vi "Main.vi"() -> ()   [LabVIEW 2026]
doc: "This Continuous Measurement sample project is based on the Queued Message Handler template.\n\nThe Event Handling Loop generates messages based on user interface actions.\n\nThe Message Handling Loop processes messages generated by the Event Handling Loop, or by other messages. There are also Acquisition and Logging message handling loop subVIs, and a chart updating loop."
uses:
  controls/Messaging Payloads/Sensor CoreData.ctl
  controls/Messaging Payloads/Sensor CoreData Cluster.ctl
  controls/UI/Units Enum.ctl
  controls/UI/Signal Enum.ctl
  controls/UI/Settings Cluster.ctl
  controls/UI/Acq Settings.ctl
  Acquisition/Instrument Specifications Configuration.ctl
  Acquisition/Instrument Specifications Cluster Configuration.ctl
  controls/UI/Measurement Role.ctl
  controls/UI/Config Settings.ctl
  Processing/Processing Settings.ctl
  Processing/Test Parameters.ctl
  Processing/Test Parameters Cluster.ctl
  controls/UI/Test Sequence Context.ctl
  controls/UI/Direction.ctl
  controls/UI/Session Identfiers.ctl
  controls/UI/Test Sequence Settings.ctl
  controls/UI/Test Sequence State.ctl
  controls/UI/Test Sequence Enum.ctl
  controls/Controller/Stimulus Settings.ctl
  controls/Controller/Stimulus Outputs.ctl
  controls/Controller/Stimulus Output.ctl
  controls/Controller/Controller Core Data.ctl
  controls/Controller/Stimulus Output Configuration.ctl
  controls/Controller/Stimulus Role.ctl
  controls/UI/UI Data.ctl
  controls/UI/UI State.ctl
  controls/UI/System Config.ctl
  controls/UI/Analog Output.ctl
  controls/UI/UUT Display Data.ctl
  Acquisition/Acquisition Payload.ctl
  Acquisition/Acquisition Context.ctl
  support/Architecture/Message Queue/Enqueue Message (Single).vi
  support/Architecture/Message Queue/Enqueue Message (Array).vi
  <vilib>/Utility/error.llb/Error Cluster From Error Code.vi
  <vilib>/ErrorRing/Error Ring.xnode
  support/Architecture/User Event - Stop/User Event - Stop.lvlib
  support/Architecture/Message Queue/Message Queue.lvlib
  Settings/Settings Dialog.vi
  Settings/Settings.lvlib
  Database/Database.lvlib
  Logging/Logging.lvlib
  Processing/Processing_Engine.lvlib
  Acquisition/Acquisition.lvlib
  support/UI Utilities/Login.vi
  Admin/Admin.lvlib
  Analysis/Analysis Dialog.vi
  Analysis/Analysis.lvlib
panel:
  in  "Manage Serial Numbers":bool
  in  "Simulation Mode":bool
  in  "Stop":bool
  in  "Start":bool
  out "Sensor Information":T1
  in  "Generate Analytics":bool
  out "Data":waveform(dbl)[](graph)
  in  "Settings":bool
  out "Status":string
  in  "Exit":bool
  # "Live Data"
  # "Test Control"
  # "ON"
  # "Automated Calibration & Test System\nMulti-Sensor Instrument Calibration Platform"
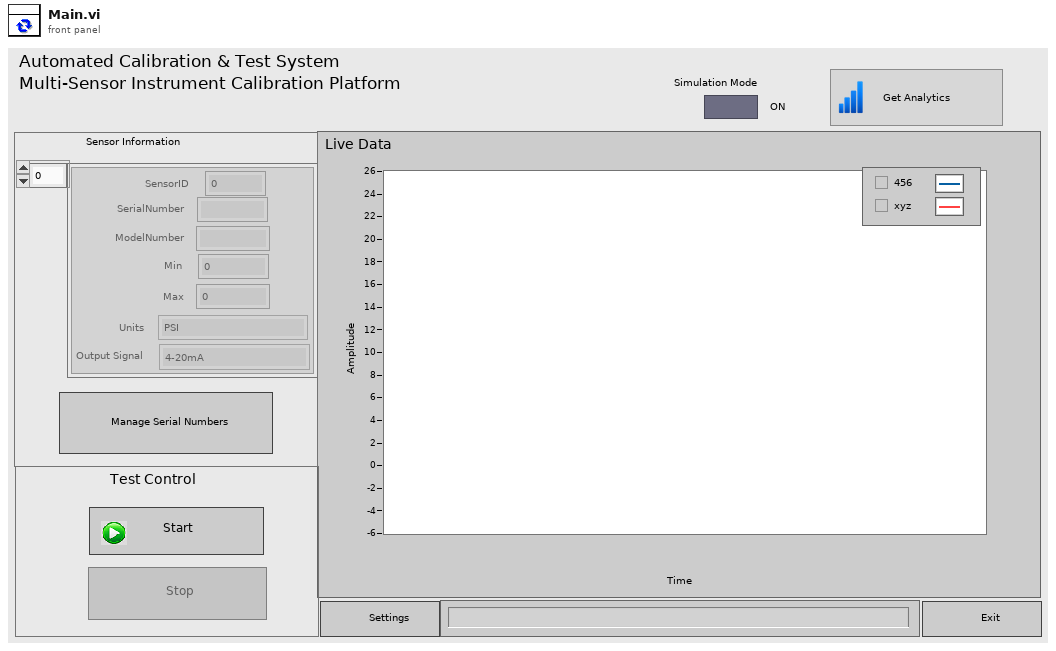
[diagram p1: front panel]
types:
  T1 = typedef "Sensor CoreData.ctl" = T2[]
  T2 = typedef "Settings.lvlib/Sensor CoreData Cluster.ctl" = cluster{"SerialNumber":string, "ModelNumber":string, "Min":dbl, "Max":dbl, "Units":T3, "Output Signal":T4, "SensorID":i32}
  T3 = typedef "Units Enum.ctl" = enum16{"PSI", "Deg C", "kPa", "GPM"}
  T4 = typedef "Signal Enum.ctl" = enum16{"4-20mA", "0-10V", "Thermocouple Type K"}
  T5 = typedef "UUT Display Data.ctl" = cluster{"Waveforms":waveform(dbl)[], "SensorIDs":i32[]}
  T6 = typedef "System Config.ctl" = cluster{"AdminHash":string, "LogFileBasePath ":path, "Config Settings":T7, "AnalogOutput":T8}
  T7 = typedef "Config Settings.ctl" = cluster{"Simulated Sensor Injection":dbl, "Base Device Name":string, "Simulation Mode":string}
  T8 = typedef "Settings.lvlib/Analog Output.ctl" = cluster{"Pressure Controller":string, "Temperature Controller":string}
  T9 = typedef "UI State.ctl" = enum16{"Idle", "Acquiring and Logging", "Waiting for Exit", "Waiting for Exit (Acq Stopped)", "Waiting for Exit (Log Stopped)", "Waiting for Stop", "Waiting for Stop (Acq Stopped)", "Waiting for Stop (Log Stopped)"}
  T10 = typedef "UI Data.ctl" = cluster{"Start Ref":refnum<vi>, "Stop Ref":refnum<vi>, "Settings Ref":refnum<vi>, "Exit Ref":refnum<vi>, "Status Ref":refnum<vi>, "Data Ref":refnum<vi>, "Sim  Refnum":refnum<vi>}
  T11 = typedef "Settings Cluster.ctl" = cluster{"Acq Settings":T12, "Processing Settings":T16, "Session Identifiers":T21, "Test Sequence Settings":T22, "Stimulus Settings":T25}
  T12 = typedef "Acq Settings.ctl" = cluster{"Instrument Specifications":T13, "Config Settings":T7}
  T13 = typedef "Acquisition.lvlib/Instrument Specifications Configuration.ctl" = T14[]
  T14 = typedef "Acquisition.lvlib/Instrument Specifications Cluster Configuration.ctl" = cluster{"Sensor ID *":i32, "Target Sample Rate (Hz) *":dbl, "Steady-State Duration (s) *":i32, "Allowed Tolerance (%) FS *":dbl, "Max Settling Timeout (s) *":i32, "Physical Channel":string, "Measurement Role":T15}
  T15 = typedef "Settings.lvlib/Measurement Role.ctl" = enum16{"Reference", "UUT"}
  T16 = typedef "Processing_Engine.lvlib/Processing Settings.ctl" = cluster{"Sensor CoreData":T1, "Test Parameters":T17, "Measurement Roles":T15[], "Test Sequence Context":T19}
  T17 = typedef "Processing_Engine.lvlib/Test Parameters.ctl" = T18[]
  T18 = typedef "Settings.lvlib/Test Parameters Cluster.ctl" = cluster{"Steady-State Duration (s)":i32, "Allowed Tolerance (%) FS":dbl, "Max Settling Timeout (s)":i32}
  T19 = typedef "Settings.lvlib/Test Sequence Context.ctl" = cluster{"Direction":T20, "Cycle Number":i32, "Setpoint":dbl}
  T20 = typedef "Settings.lvlib/Direction.ctl" = enum16{"Acsending", "Descending"}
  T21 = typedef "Session Identfiers.ctl" = cluster{"SerialNumber":string[], "OperatorName":string}
  T22 = typedef "Test Sequence Settings.ctl" = cluster{"Test Sequence State":T23}
  T23 = typedef "Settings.lvlib/Test Sequence State.ctl" = cluster{"Test Sequence Enum":T24, "Point Index":i32, "Current Target":dbl, "Previous Target":dbl, "Simulation?":bool, "Direction":T20, "Transition Active?":bool, "Cycle Number":i32}
  T24 = typedef "Test Sequence Enum.ctl" = enum16{"Idle", "Start Point", "Point Complete", "Test Complete", "Abort Test", "Reset"}
  T25 = typedef "Settings.lvlib/Stimulus Settings.ctl" = cluster{"Stimulus Outputs":T26}
  T26 = typedef "Settings.lvlib/Stimulus Outputs.ctl" = T27[]
  T27 = typedef "Settings.lvlib/Stimulus Output.ctl" = cluster{"Controller Core Data":T28, "Stimulus Output Configuration":T29}
  T28 = typedef "Settings.lvlib/Controller Core Data.ctl" = cluster{"Min":dbl, "Max":dbl, "Units":T3, "Input Signal Type":T4, "Input Signal Min":dbl, "Input Signal Max":dbl}
  T29 = typedef "Settings.lvlib/Stimulus Output Configuration.ctl" = cluster{"DAQmx AO Physical Channel":tag, "Role":T30, "Model Numbers":string, "Serial Numbers":string, "Row":i32}
  T30 = typedef "Stimulus Role.ctl" = enum16{"Pressure Controller", "Temperature Controller"}
  T31 = typedef "Message Queue.lvlib/All Message Queues.ctl" = cluster{"UI":refnum<queue>, "Database":refnum<queue>, "Processing":refnum<queue>, "Acquisition":refnum<queue>, "Logging":refnum<queue>, "Analysis":refnum<queue>}
  T32 = enum8{"Enabled", "Disabled", "Disabled and Grayed Out"}
  T33 = typedef "Acquisition.lvlib/Acquisition Payload.ctl" = cluster{"Acq Settings":T12, "Acquisition Context":T34, "Stimulus Settings":T25}
  T34 = typedef "Acquisition.lvlib/Acquisition Context.ctl" = cluster{"Setpoint":dbl, "Previous Setpoint":dbl, "Transition Start Time":dbl, "Transition Active?":bool, "Acknowledgement Pending?":bool}
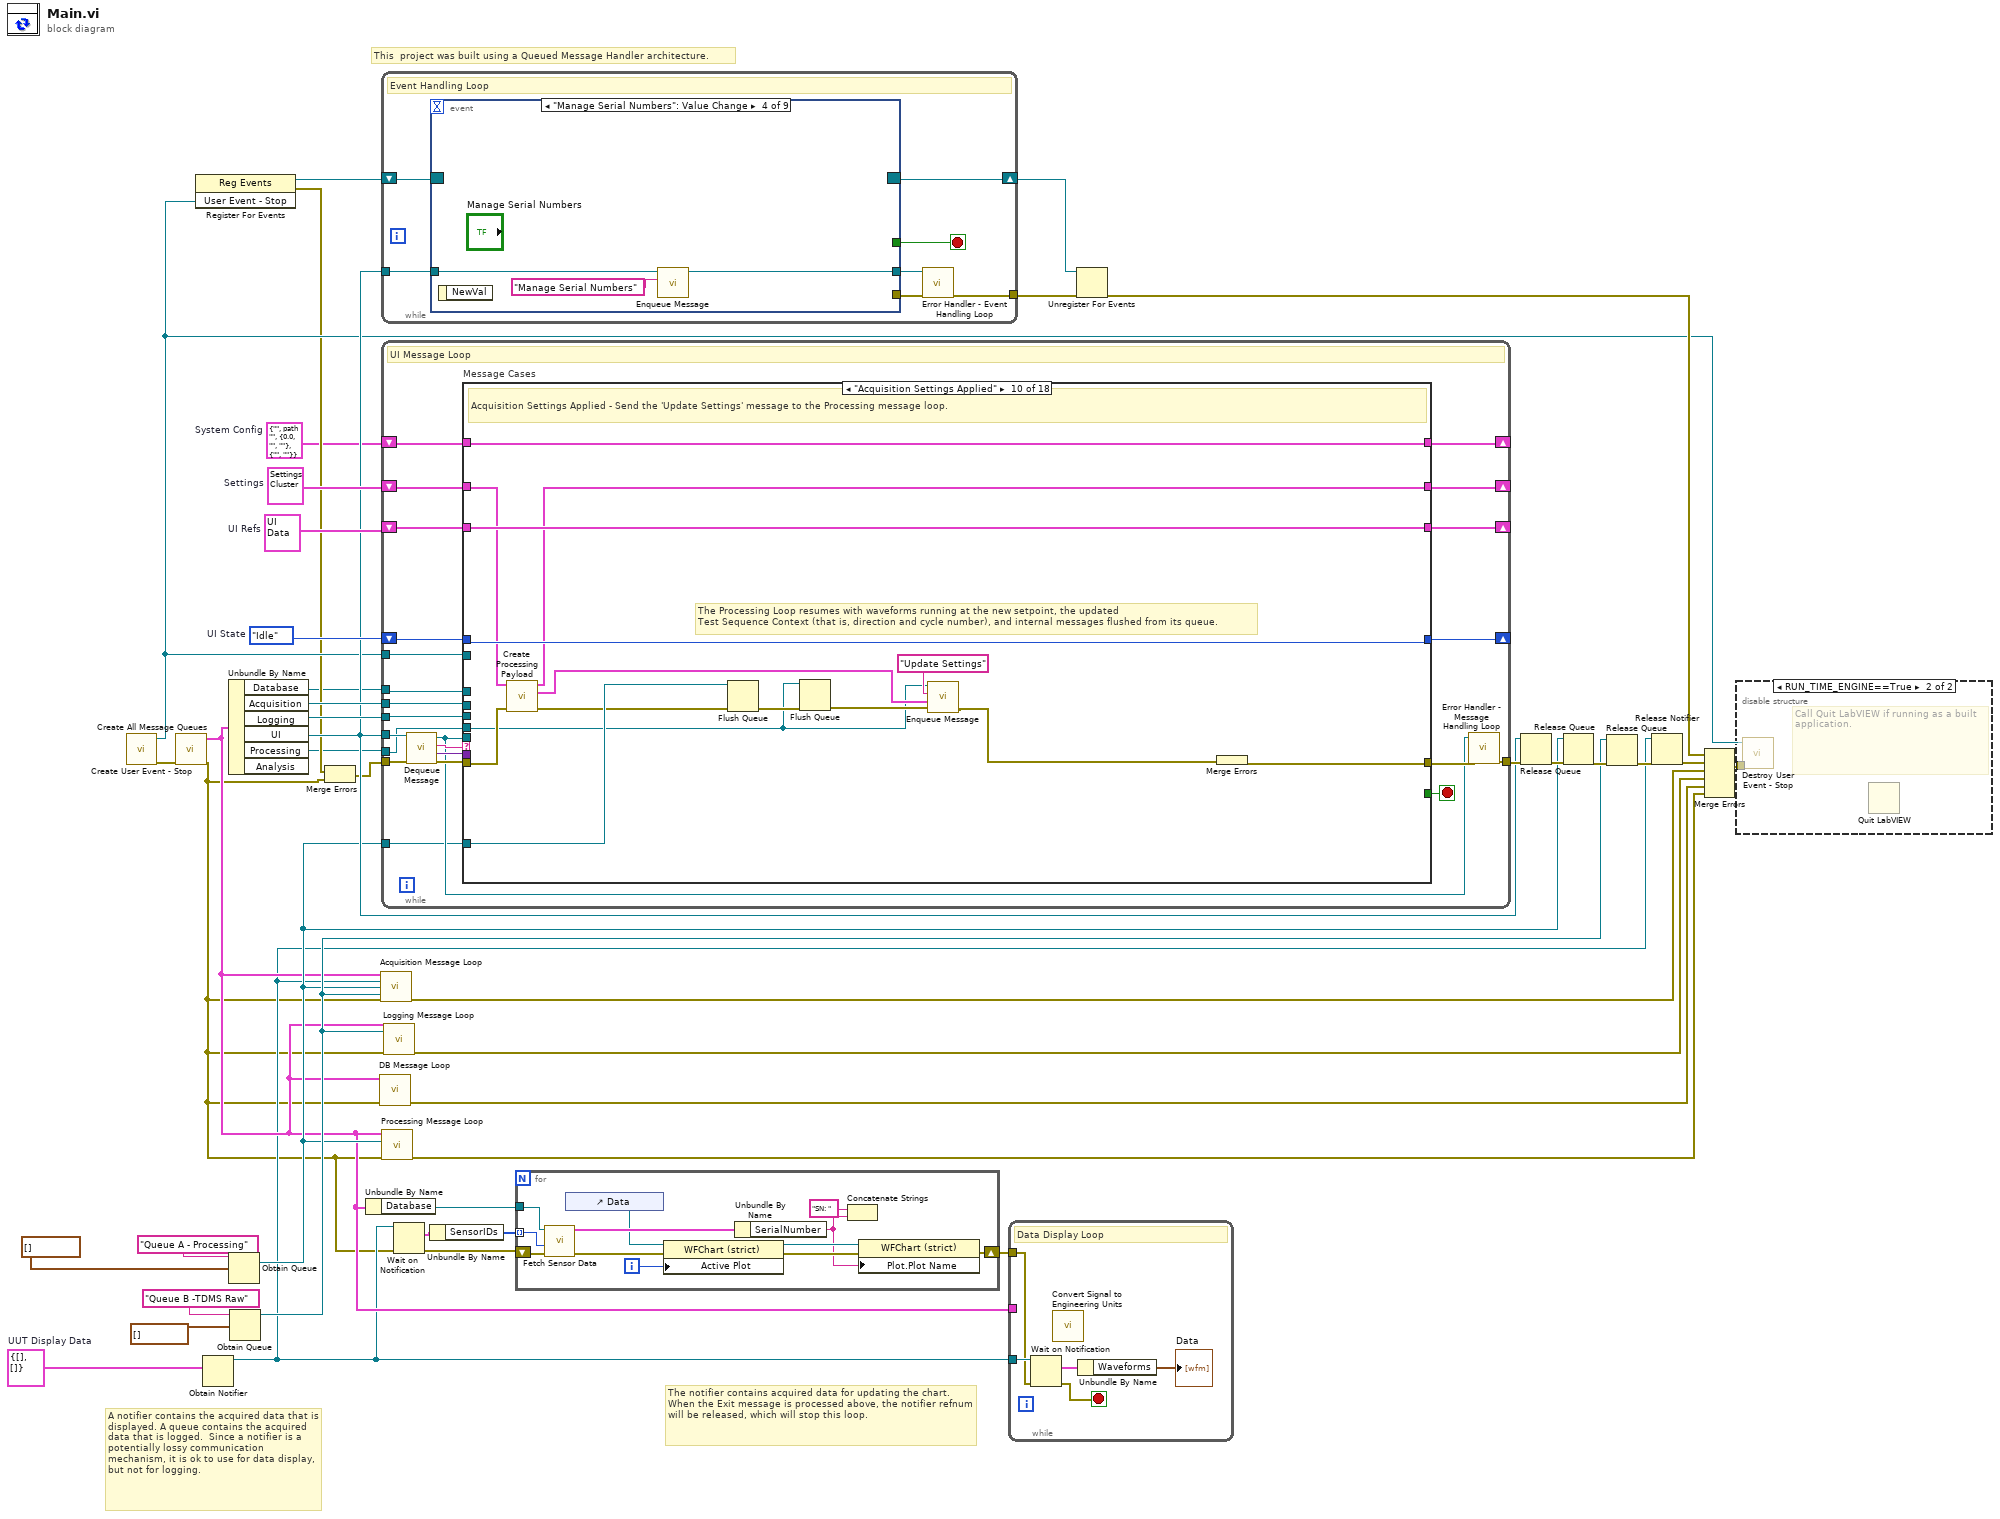
[diagram p0: block diagram]
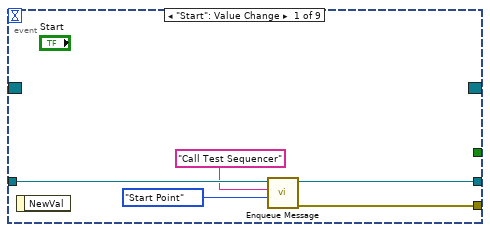
[diagram p3: hidden frame]
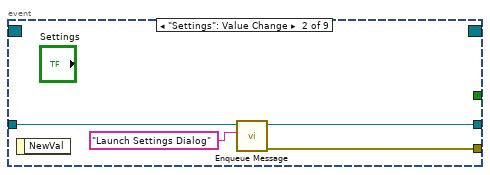
[diagram p4: hidden frame]
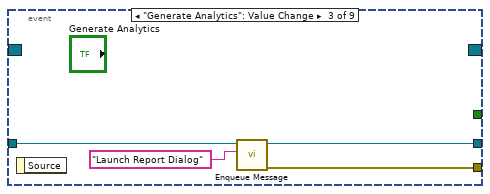
[diagram p5: hidden frame]
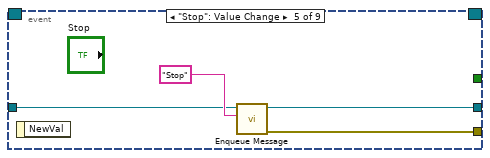
[diagram p6: hidden frame]
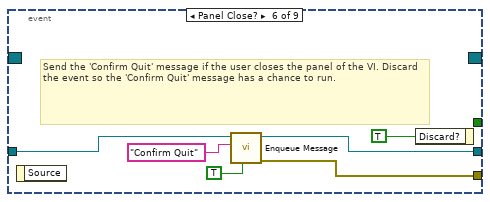
[diagram p7: hidden frame]
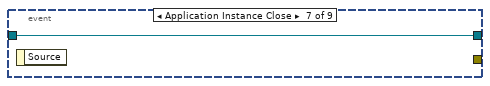
[diagram p8: hidden frame]
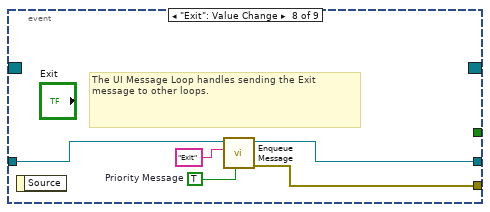
[diagram p9: hidden frame]
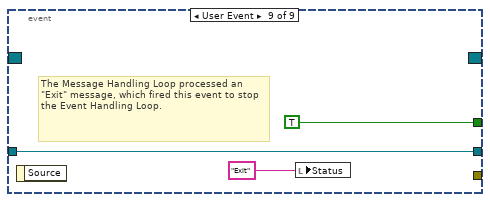
[diagram p10: hidden frame]
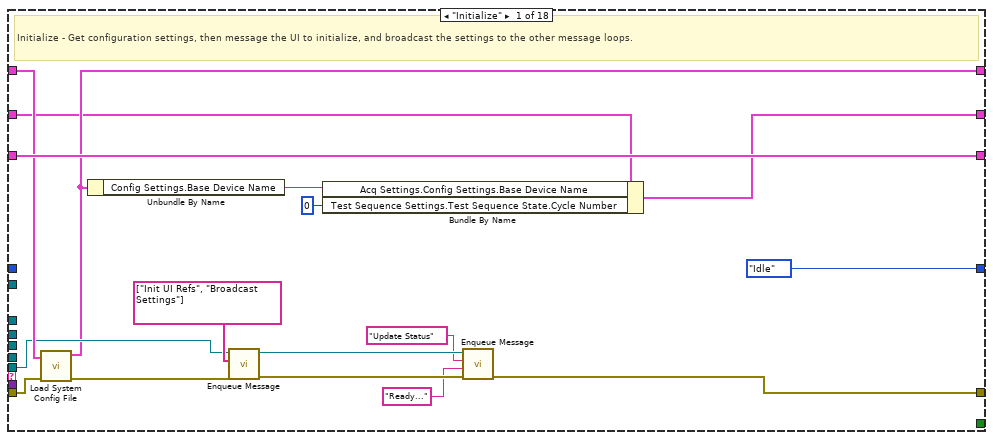
[diagram p11: hidden frame]
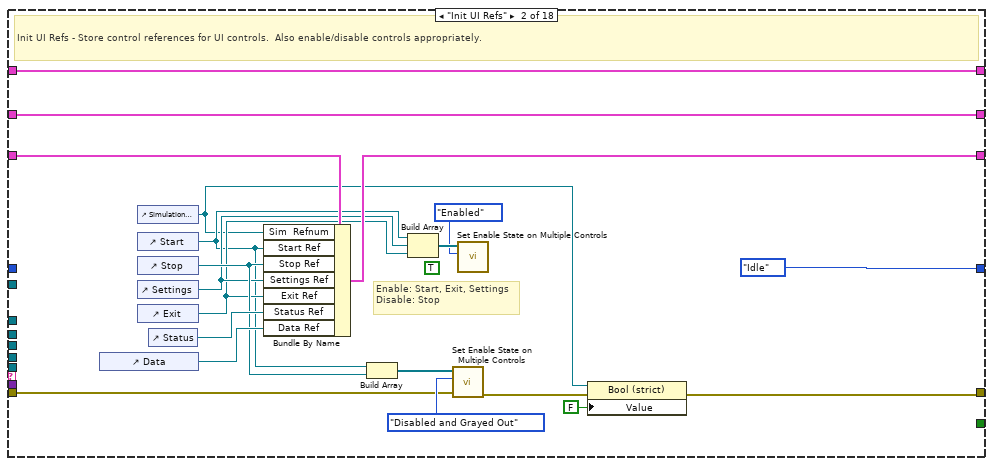
[diagram p12: hidden frame]
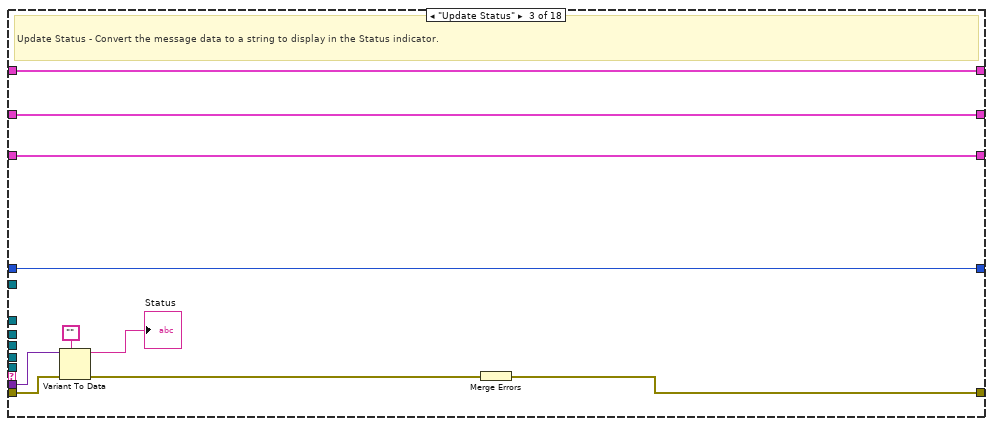
[diagram p13: hidden frame]
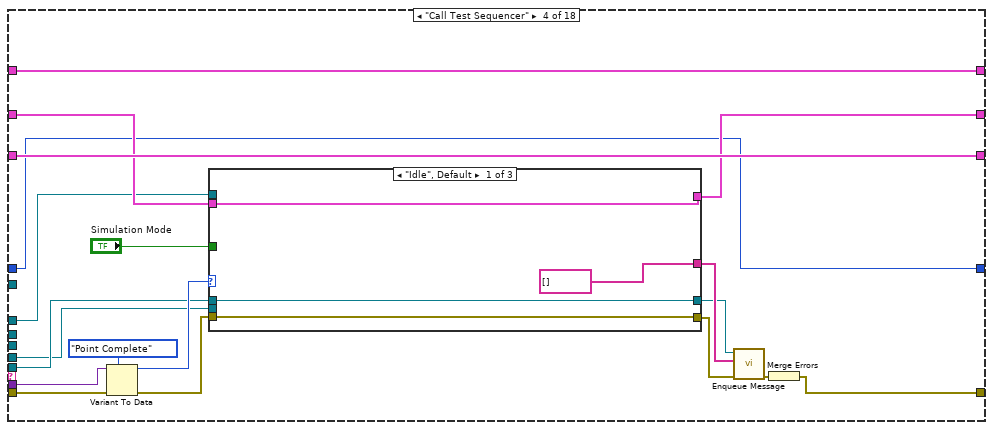
[diagram p14: hidden frame]
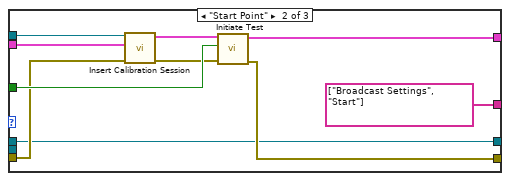
[diagram p15: hidden frame]
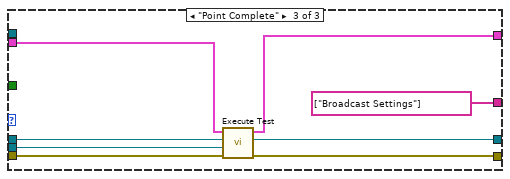
[diagram p16: hidden frame]
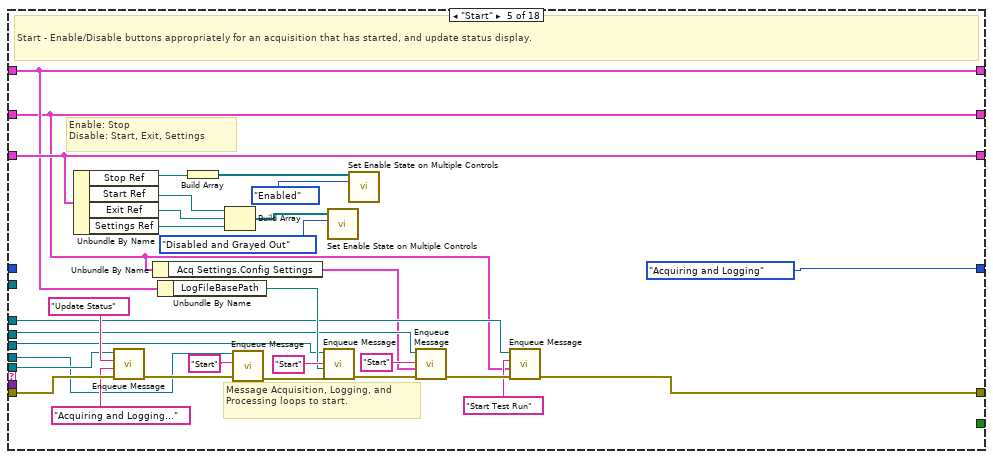
[diagram p17: hidden frame]
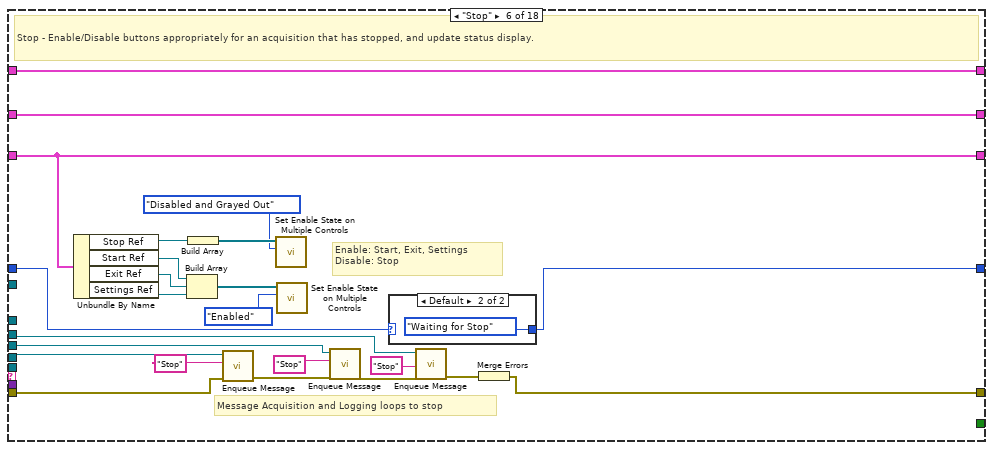
[diagram p18: hidden frame]
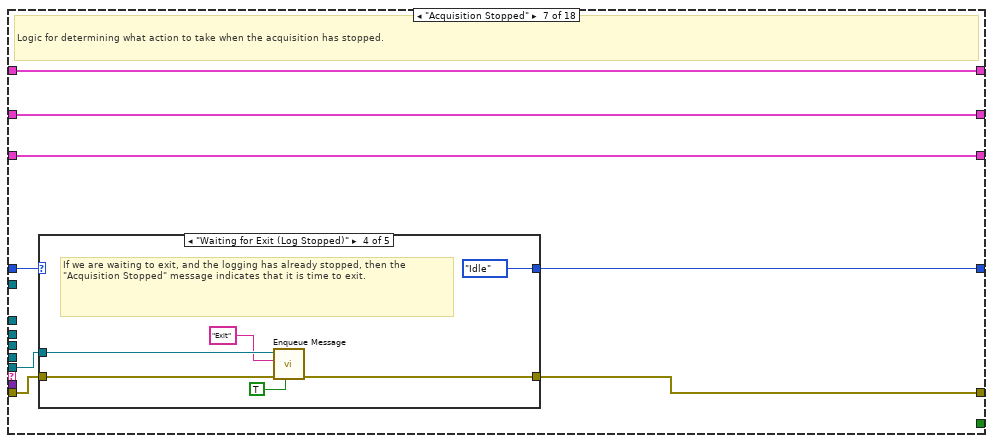
[diagram p20: hidden frame]
diagram:
  w9 = T5 {"Waveforms"=[], "SensorIDs"=[]}  # UUT Display Data
  w20 = T6 {"AdminHash"="", "LogFileBasePath "=path "", "Config Settings"={"Simulated Sensor Injection"=0.0, "Base Device Name"="", "Simulation Mode"=""}, "AnalogOutput"={"Pressure Controller"="", "Temperature Controller"=""}}  # System Config
  w32 = UI_State."Idle"  # UI State
  w35 = T10 {"Start Ref"=refnum, "Stop Ref"=refnum, "Settings Ref"=refnum, "Exit Ref"=refnum, "Status Ref"=refnum, "Data Ref"=refnum, "Sim  Refnum"=refnum}  # UI Refs
  w38 = T11 {"Acq Settings"={"Instrument Specifications"=[], "Config Settings"={"Simulated Sensor Injection"=0.0, "Base Device Name"="", "Simulation Mode"=""}}, "Processing Settings"={"Sensor CoreData"=[], "Test Parameters"=[], "Measurement Roles"=[], "Test Sequence Context"={"Direction"=enum."Acsending", "Cycle Number"=0, "Setpoint"=0.0}}, "Session Identifiers"={"SerialNumber"=[], "OperatorName"=""}, "Test Sequence Settings"={"Test Sequence State"={"Test Sequence Enum"=enum."Idle", "Point Index"=0, "Current Target"=0.0, "Previous Target"=0.0, "Simulation?"=FALSE, "Direction"=enum."Acsending", "Transition Active?"=FALSE, "Cycle Number"=0}}, "Stimulus Settings"={"Stimulus Outputs"=[]}}  # Settings
  # "This  project was built using a Queued Message Handler architecture."
  # "A notifier contains the acquired data that is displayed. A queue contains the acquired data that is logged.  Since a notifier is a potentially lossy communication mechanism, it is ok to use for data display, but not for logging."
  # "The notifier contains acquired data for updating the chart. When the Exit message is processed above, the notifier refnum will be released, which will stop this loop."
  n1 = call "Create User Event - Stop.vi"() -> ("error out"=w40:errorcluster, "User Event - Stop"=w25:refnum<user-event>)  [unwired: 10 in]
  n2 = call "Create All Message Queues.vi"("error in (no error)"=w40) -> ("error out"=w2:errorcluster, "Message Queues out"=w6:T31)  [unwired: 9 in]
  n3 = register-events(w25) -> (reference out=w26:refnum<event-registration>, error out=w23:errorcluster)  [unwired: 2 in]
  n4 = Obtain Notifier(notification data type=w9) -> (notifier out=w4:refnum<notifier>)  [unwired: 3 in, 2 out]
  n5 = Unbundle By Name(w6) -> ("Database"=w21:refnum<queue>, "Acquisition"=w34:refnum<queue>, "Logging"=w33:refnum<queue>, "UI"=w30:refnum<queue>, "Processing"=w19:refnum<queue>)  [unwired: 1 out]
  n6 = Obtain Queue(name (unnamed)="Queue A - Processing", element data type=waveform(dbl)[] []) -> (queue out=w10:refnum<queue>)  [unwired: 3 in, 2 out]
  n7 = Obtain Queue(name (unnamed)="Queue B -TDMS Raw", element data type=waveform(dbl)[] []) -> (queue out=w11:refnum<queue>)  [unwired: 3 in, 2 out]
  n8 = Merge Errors(w23, w2) -> (w24:errorcluster)
  n9 = Unbundle By Name(w6) -> ("Database"=w7:refnum<queue>)
  n10 = call "DB Message Loop.vi"("error in (no error)"=w2, "Message Queues"=w6) -> ("error out"=w22:errorcluster)  [unwired: 9 in]
  n11 = call "Acquisition Message Loop.vi"("Message Queues"=w6, "Data Notifier"=w4, "Queue A - Processing"=w10, "Queue B -TDMS Raw"=w11, "error in (no error)"=w2) -> ("error out"=w41:errorcluster)  [unwired: 10 in]
  n12 = while {
    tunnel: w30 -> [w49]
    tunnel: [w46] -> w42
    shift-right: [w48] -> w36
    shift-left: w26 -> [w50]
    stop <- w47 stop-if-true
    # "Event Handling Loop"
    n13 = event shown="[3] \"Manage Serial Numbers\": Value Change" {
      selector: w50 -> [_ _ _ _ _ _ _ _ _]
      dyn-events: [_ _ _ _ _ _ _ _ _] -> w48
      timeout: _ -> [_ _ _ _ _ _ _ _ _]
      tunnel: [_ _ _ _ _ _ _ _ TRUE ("Discard?")] -> w47
      tunnel: w49 -> [w55 w58 w62 w65 w69 w74 w77 w79 w83]
      tunnel: [w53 w56 w60 _ w68 w72 _ w82 _] -> w45
      tunnel: [w52 w57 w61 w64 w67 w73 w77 w78 w83] -> w44
      event "Start": Value Change {
        n14 = event-data() -> ()  [unwired: 1 in, 1 out]
        n15 = call-poly "Enqueue Message.vi"("Message Data"=Test_Sequence_Enum."Start Point" ("Test Sequence State.Test Sequence Enum"), "Message"="Call Test Sequencer", "Message Queue"=w55) -> ("error out"=w53:errorcluster, "dup Message Queue"=w52:refnum<queue>)  [unwired: 7 in]
      }
      event "Settings": Value Change {
        n16 = event-data() -> ()  [unwired: 1 in, 1 out]
        n17 = call-poly "Enqueue Message.vi"("Message"="Launch Settings Dialog", "Message Queue"=w58) -> ("error out"=w56:errorcluster, "dup Message Queue"=w57:refnum<queue>)  [unwired: 8 in]
      }
      event "Generate Analytics": Value Change {
        n18 = event-data() -> ()  [unwired: 1 in, 1 out]
        n19 = call-poly "Enqueue Message.vi"("Message"="Launch Report Dialog", "Message Queue"=w62) -> ("error out"=w60:errorcluster, "dup Message Queue"=w61:refnum<queue>)  [unwired: 8 in]
      }
      event "Manage Serial Numbers": Value Change {
        n20 = event-data() -> ()  [unwired: 1 in, 1 out]
        n21 = call-poly "Enqueue Message.vi"("Message"="Manage Serial Numbers", "Message Queue"=w65) -> ("dup Message Queue"=w64:refnum<queue>)  [unwired: 8 in, 1 out]
      }
      event "Stop": Value Change {
        n22 = event-data() -> ()  [unwired: 1 in, 1 out]
        n23 = call-poly "Enqueue Message.vi"("Message"="Stop", "Message Queue"=w69) -> ("error out"=w68:errorcluster, "dup Message Queue"=w67:refnum<queue>)  [unwired: 8 in]
      }
      event Panel Close? {
        # "Send the 'Confirm Quit' message if the user closes the panel of the VI. Discard the event so the 'Confirm Quit' message has a chance to run."
        n24 = event-data() -> ()  [unwired: 1 in, 1 out]
        n25 = call-poly "Enqueue Message.vi"("Priority Message? (F)"=TRUE, "Message"="Confirm Quit", "Message Queue"=w74) -> ("error out"=w72:errorcluster, "dup Message Queue"=w73:refnum<queue>)  [unwired: 7 in]
        n26 = event-data("Discard?"=TRUE) -> ()  [unwired: 1 in, 1 out]
      }
      event Application Instance Close {
        n27 = event-data() -> ()  [unwired: 1 in, 1 out]
      }
      event "Exit": Value Change {
        w80 = TRUE  # Priority Message
        # "The UI Message Loop handles sending the Exit message to other loops."
        n28 = event-data() -> ()  [unwired: 1 in, 1 out]
        n29 = call-poly "Enqueue Message.vi"("Priority Message? (F)"=w80, "Message"="Exit", "Message Queue"=w79) -> ("error out"=w82:errorcluster, "dup Message Queue"=w78:refnum<queue>)  [unwired: 7 in]
      }
      event User Event {
        # "The Message Handling Loop processed an \"Exit\" message, which fired this event to stop the Event Handling Loop."
        n30 = event-data() -> ()  [unwired: 1 in, 1 out]
        n31 = local write "Status"("Exit" ("Exit String")) -> ()
      }
    }
    n32 = call "Error Handler - Event Handling Loop.vi"("error in (no error)"=w45, "Message Queue"=w44) -> ("dup error in"=w46:errorcluster)  [unwired: 8 in, 1 out]
  }
  n33 = while {
    tunnel: w30 -> [w102]
    tunnel: w25 -> [w107]
    shift-right: [w101] -> _
    shift-left: w38 -> [w100]
    shift-right: [w98] -> _
    shift-left: w35 -> [w99]
    tunnel: w34 -> [w97]
    tunnel: w33 -> [w96]
    shift-right: [w91] -> _
    shift-left: w32 -> [w92]
    tunnel: w24 -> [w106]
    tunnel: [w95] -> w43
    tunnel: w21 -> [w90]
    shift-right: [w88] -> _
    shift-left: w20 -> [w89]
    tunnel: w19 -> [w87]
    tunnel: w10 -> [w86]
    stop <- w108 stop-if-true
    # "UI Message Loop"
    n34 = call "Dequeue Message.vi"("error in (no error)"=w106, "Message Queue"=w102) -> ("error out"=w105:errorcluster, "Message Data"=w103:variant, "Message"=w104:string, "dup Message Queue"=w93:refnum<queue>)  [unwired: 6 in]
    n35 = case "Message Cases" shown="\"Acquisition Settings Applied\"" w104 {
      selector: w104 -> [_ _ _ _ _ _ _ _ _ _ _ _ _ _ _ _ _ w470]
      tunnel: w93 -> [w116 _ _ w159 w204 _ w257 w283 _ _ w350 _ w400 _ w416 _ _ _]
      tunnel: w105 -> [w118 w131 w154 w174 w227 w229 w258 w284 w306 w330 w358 w391 w401 w403 w415 w447 w467 _]
      tunnel: [w110 w127 w155 w168 w207 w233 w255 w281 w320 w335 w341 w387 w396 w406 w414 w459 w466 w469] -> w94
      tunnel: [_ _ _ _ _ _ _ _ _ _ _ _ _ _ _ TRUE _ _] -> w108
      tunnel: w103 -> [_ _ w153 w173 _ _ _ _ _ _ _ _ _ w407 _ w452 _ _]
      tunnel: w107 -> [_ _ _ _ _ _ _ _ _ _ _ _ _ _ _ w460 _ _]
      tunnel: [w111 w145 w149 w169 w198 w251 w261 w287 w307 w327 w351 w386 w393 w411 w419 w458 w465 w473] -> w101
      tunnel: w100 -> [w112 w145 w149 w167 w198 w251 w261 w287 w307 w329 w355 w386 w393 w411 w419 w458 w465 w473]
      tunnel: w99 -> [w121 w144 w148 w172 w225 w250 w260 w286 w319 w334 w345 w390 w398 w410 w418 w457 w464 w472]
      tunnel: [w121 w141 w148 w172 w225 w250 w260 w286 w319 w334 w345 w390 w398 w410 w418 w457 w464 w472] -> w98
      tunnel: w97 -> [_ _ _ _ w203 w240 _ _ w314 _ _ _ _ _ _ w449 _ _]
      tunnel: w96 -> [_ _ _ _ w202 w230 _ _ _ _ _ _ _ _ _ w456 _ _]
      tunnel: w92 -> [_ _ w147 w166 _ w237 w259 w285 w318 w333 w357 w389 w397 w405 w417 _ w463 w471]
      tunnel: [UI_State."Idle" ("UI State") UI_State."Idle" ("UI State") w147 w166 UI_State."Acquiring and Logging" ("UI State") w238 w256 w282 w318 w333 w357 w389 w397 w405 w413 UI_State."Idle" ("UI State") w463 w471] -> w91
      tunnel: w90 -> [_ _ _ w157 w205 _ _ _ _ _ w356 w385 w392 _ _ w450 _ _]
      tunnel: w89 -> [w117 w134 w146 w171 w214 w236 w254 w280 w317 w332 w354 w388 w395 w402 w412 w446 w462 w468]
      tunnel: [w113 w134 w146 w171 w214 w236 w254 w280 w317 w332 w354 w388 w395 w402 w412 w446 w462 w468] -> w88
      tunnel: w87 -> [_ _ _ w156 w201 w231 _ _ _ w321 _ _ _ _ _ w441 _ _]
      tunnel: w86 -> [_ _ _ _ _ _ _ _ _ w325 _ _ _ _ _ _ _ _]
      frame "Initialize" {
        # "Initialize - Get configuration settings, then message the UI to initialize, and broadcast the settings to the other message loops."
        n36 = call "Load System Config File.vi"("error in (no error)"=w118, "System Config in"=w117) -> ("error out"=w115:errorcluster, "System Config out"=w113:T6)  [unwired: 8 in]
        n37 = Unbundle By Name(w113) -> ("Config Settings.Base Device Name"=w114:string)
        n38 = call-poly "Enqueue Message.vi"("error in (no error)"=w115, "Message Array"=string[] ["Init UI Refs", "Broadcast Settings"], "Message Queue"=w116) -> ("error out"=w125:errorcluster, "dup Message Queue"=w124:refnum<queue>)  [unwired: 7 in]
        n39 = Bundle By Name(cluster=w112, "Acq Settings.Config Settings.Base Device Name"=w114, "Test Sequence Settings.Test Sequence State.Cycle Number"=0) -> (w111:T11)
        n40 = call-poly "Enqueue Message.vi"("error in (no error)"=w125, "Message Data"="Ready..." ("Ready..."), "Message"="Update Status", "Message Queue"=w124) -> ("error out"=w110:errorcluster)  [unwired: 6 in, 1 out]
      }
      frame "Init UI Refs" {
        (unwired) TRUE ("Enable?")
        # "Enable: Start, Exit, Settings\nDisable: Stop"
        # "Init UI Refs - Store control references for UI controls.  Also enable/disable controls appropriately."
        n41 = control-ref of="Data"() -> (w142:refnum<vi>)
        n42 = control-ref of="Simulation Mode"() -> (w129:refnum<vi>)
        n43 = control-ref of="Start"() -> (w130:refnum<vi>)
        n44 = control-ref of="Stop"() -> (w138:refnum<vi>)
        n45 = control-ref of="Settings"() -> (w137:refnum<vi>)
        n46 = control-ref of="Exit"() -> (w136:refnum<vi>)
        n47 = control-ref of="Status"() -> (w143:refnum<vi>)
        n48 = Bundle By Name(cluster=w144, "Sim  Refnum"=w129, "Start Ref"=w130, "Stop Ref"=w138, "Settings Ref"=w137, "Exit Ref"=w136, "Status Ref"=w143, "Data Ref"=w142) -> (w141:T10)
        n49 = Build Array(w130, w138) -> (w139:refnum<vi>[])
        n50 = Build Array(w130, w137, w136) -> (w140:refnum<vi>[])
        n51 = call "Set Enable State on Multiple Controls.vi"("Controls"=w139, "Disabled"=T32."Disabled and Grayed Out", "error in (no error)"=w131) -> ("error out"=w128:errorcluster)  [unwired: 7 in]
        n52 = call "Set Enable State on Multiple Controls.vi"("Controls"=w140, "Disabled"=T32."Enabled") -> ()  [unwired: 8 in, 1 out]
        n53 = property class="Bool (strict)"(reference=w129, error in=w128, "Value"=FALSE) -> (error out=w127:errorcluster)  [unwired: 1 out]
      }
      frame "Update Status" {
        # "Update Status - Convert the message data to a string to display in the Status indicator."
        n54 = Variant To Data(error in=w154, type="", Variant=w153) -> (data=→"Status":string, error out=w151:errorcluster)
        n55 = Merge Errors(w151) -> (w155:errorcluster)
      }
      frame "Call Test Sequencer" {
        n56 = Variant To Data(error in=w174, type=Test_Sequence_Enum."Point Complete" ("Test Sequence Enum"), Variant=w173) -> (data=w161:T24, error out=w170:errorcluster)
        n57 = case shown="\"Idle\", Default" w161 {
          tunnel: w170 -> [w177 w184 w195]
          tunnel: [w177 w188 w194] -> w164
          tunnel: [w178 w187 w193] -> w169
          tunnel: "Simulation Mode" -> [_ w186 _]
          tunnel: w167 -> [w178 w180 w192]
          tunnel: [string[] [] string[] ["Broadcast Settings", "Start"] string[] ["Broadcast Settings"]] -> w163
          tunnel: w159 -> [w175 w182 w191]
          tunnel: [w175 w182 w190] -> w158
          tunnel: w157 -> [_ w179 _]
          tunnel: w156 -> [_ _ w189]
          frame "Idle", Default {
          }
          frame "Start Point" {
            n58 = call "Insert Calibration Session.vi"("error in (no error)"=w184, "Settings in"=w180, "Database"=w179) -> ("error out"=w183:errorcluster, "Settings out"=w181:T11)  [unwired: 7 in]
            n59 = call "Initiate Test.vi"("error in (no error)"=w183, "Simulation?"=w186, "Settings in"=w181) -> ("error out"=w188:errorcluster, "Settings out"=w187:T11)  [unwired: 7 in]
          }
          frame "Point Complete" {
            n60 = call "Execute Test.vi"("error in (no error)"=w195, "Processing"=w189, "UI in"=w191, "Settings in"=w192) -> ("error out"=w194:errorcluster, "UI out"=w190:refnum<queue>, "Settings out"=w193:T11)  [unwired: 5 in]
          }
        }
        n61 = call-poly "Enqueue Message.vi"("error in (no error)"=w164, "Message Array"=w163, "Message Queue"=w158) -> ("error out"=w165:errorcluster)  [unwired: 7 in, 1 out]
        n62 = Merge Errors(w165) -> (w168:errorcluster)
      }
      frame "Start" {
        # "Message Acquisition, Logging, and \nProcessing loops to start."
        # "Enable: Stop\nDisable: Start, Exit, Settings"
        # "Start - Enable/Disable buttons appropriately for an acquisition that has started, and update status display."
        n63 = Unbundle By Name(w225) -> ("Stop Ref"=w222:refnum<vi>, "Start Ref"=w221:refnum<vi>, "Exit Ref"=w220:refnum<vi>, "Settings Ref"=w219:refnum<vi>)
        n64 = call-poly "Enqueue Message.vi"("error in (no error)"=w227, "Message Data"="Acquiring and Logging..." ("Acquiring and Logging..."), "Message"="Update Status", "Message Queue"=w204) -> ("error out"=w210:errorcluster)  [unwired: 6 in, 1 out]
        n65 = Unbundle By Name(w198) -> ("Acq Settings.Config Settings"=w197:T7)
        n66 = Unbundle By Name(w214) -> ("LogFileBasePath"=w213:path)
        n67 = Build Array(w222) -> (w223:refnum<vi>[])
        n68 = Build Array(w221, w220, w219) -> (w224:refnum<vi>[])
        n69 = call-poly "Enqueue Message.vi"("error in (no error)"=w210, "Message"="Start", "Message Queue"=w201) -> ("error out"=w209:errorcluster)  [unwired: 7 in, 1 out]
        n70 = call-poly "Enqueue Message.vi"("error in (no error)"=w209, "Message Data"=w213, "Message"="Start", "Message Queue"=w202) -> ("error out"=w217:errorcluster)  [unwired: 6 in, 1 out]
        n71 = call "Set Enable State on Multiple Controls.vi"("Controls"=w224, "Disabled"=T32."Disabled and Grayed Out") -> ()  [unwired: 8 in, 1 out]
        n72 = call "Set Enable State on Multiple Controls.vi"("Controls"=w223, "Disabled"=T32."Enabled") -> ()  [unwired: 8 in, 1 out]
        n73 = call-poly "Enqueue Message.vi"("error in (no error)"=w217, "Message Data"=w197, "Message"="Start", "Message Queue"=w203) -> ("error out"=w208:errorcluster)  [unwired: 6 in, 1 out]
        n74 = call-poly "Enqueue Message.vi"("error in (no error)"=w208, "Message Data"=w198, "Message"="Start Test Run", "Message Queue"=w205) -> ("error out"=w207:errorcluster)  [unwired: 6 in, 1 out]
      }
      frame "Stop" {
        # "Message Acquisition and Logging loops to stop"
        # "Enable: Start, Exit, Settings\nDisable: Stop"
        # "Stop - Enable/Disable buttons appropriately for an acquisition that has stopped, and update status display."
        n75 = Unbundle By Name(w250) -> ("Stop Ref"=w247:refnum<vi>, "Start Ref"=w246:refnum<vi>, "Exit Ref"=w245:refnum<vi>, "Settings Ref"=w244:refnum<vi>)
        n76 = Build Array(w246, w245, w244) -> (w249:refnum<vi>[])
        n77 = Build Array(w247) -> (w248:refnum<vi>[])
        n78 = call-poly "Enqueue Message.vi"("error in (no error)"=w229, "Message"="Stop", "Message Queue"=w231) -> ("error out"=w228:errorcluster)  [unwired: 7 in, 1 out]
        n79 = call "Set Enable State on Multiple Controls.vi"("Controls"=w248, "Disabled"=T32."Disabled and Grayed Out") -> ()  [unwired: 8 in, 1 out]
        n80 = call "Set Enable State on Multiple Controls.vi"("Controls"=w249, "Disabled"=T32."Enabled") -> ()  [unwired: 8 in, 1 out]
        n81 = call-poly "Enqueue Message.vi"("error in (no error)"=w228, "Message"="Stop", "Message Queue"=w230) -> ("error out"=w242:errorcluster)  [unwired: 7 in, 1 out]
        n82 = case shown="Default" w237 {
          selector: w237 -> [w252 _]
          tunnel: [w252 UI_State."Waiting for Stop" ("UI State")] -> w238
          frame "Waiting for Exit" {
          }
          frame Default {
          }
        }
        n83 = call-poly "Enqueue Message.vi"("error in (no error)"=w242, "Message"="Stop", "Message Queue"=w240) -> ("error out"=w241:errorcluster)  [unwired: 7 in, 1 out]
        n84 = Merge Errors(w241) -> (w233:errorcluster)
      }
      frame "Acquisition Stopped" {
        # "Logic for determining what action to take when the acquisition has stopped."
        n85 = case shown="\"Waiting for Exit (Log Stopped)\"" w259 {
          selector: w259 -> [w263 _ _ _ _]
          tunnel: w258 -> [w262 w265 w267 w273 w279]
          tunnel: w257 -> [_ _ _ w271 w276]
          tunnel: [w263 UI_State."Waiting for Exit (Acq Stopped)" ("UI State") UI_State."Waiting for Stop (Acq Stopped)" ("UI State") UI_State."Idle" ("UI State") UI_State."Idle" ("UI State")] -> w256
          tunnel: [w262 w265 w267 w272 w277] -> w255
          frame Default {
          }
          frame "Waiting for Exit", "Waiting for Exit (Acq Stopped)" {
          }
          frame "Waiting for Stop", "Waiting for Stop (Acq Stopped)" {
          }
          frame "Waiting for Exit (Log Stopped)" {
            # "If we are waiting to exit, and the logging has already stopped, then the \"Acquisition Stopped\" message indicates that it is time to exit."
            n86 = call-poly "Enqueue Message.vi"("Priority Message? (F)"=TRUE, "error in (no error)"=w273, "Message"="Exit", "Message Queue"=w271) -> ("error out"=w272:errorcluster)  [unwired: 6 in, 1 out]
          }
          frame "Waiting for Stop (Log Stopped)" {
            # "If we are waiting to stop, and the logging has already stopped, then the \"Acquisition Stopped\" message indicates that it is time to stop."
            n87 = call-poly "Enqueue Message.vi"("error in (no error)"=w279, "Message Data"="Ready..." ("Ready..."), "Message"="Update Status", "Message Queue"=w276) -> ("error out"=w277:errorcluster)  [unwired: 6 in, 1 out]
          }
        }
      }
      frame "Logging Stopped" {
        # "Logic for determining what action to take when the logging has stopped."
        n88 = case shown="Default" w285 {
          selector: w285 -> [w289 _ _ _ _]
          tunnel: w284 -> [w288 w291 w293 w299 w302]
          tunnel: w283 -> [_ _ _ w297 w301]
          tunnel: [w289 UI_State."Waiting for Exit (Log Stopped)" ("UI State") UI_State."Waiting for Stop (Log Stopped)" ("UI State") UI_State."Idle" ("UI State") UI_State."Idle" ("UI State")] -> w282
          tunnel: [w288 w291 w293 w298 w300] -> w281
          frame Default {
          }
          frame "Waiting for Exit", "Waiting for Exit (Log Stopped)" {
          }
          frame "Waiting for Stop", "Waiting for Stop (Log Stopped)" {
          }
          frame "Waiting for Exit (Acq Stopped)" {
            # "If we are waiting to exit, and the acquisition has already stopped, then the \"Logging Stopped\" message indicates that it is time to exit."
            n89 = call-poly "Enqueue Message.vi"("Priority Message? (F)"=TRUE, "error in (no error)"=w299, "Message"="Exit", "Message Queue"=w297) -> ("error out"=w298:errorcluster)  [unwired: 6 in, 1 out]
          }
          frame "Waiting for Stop (Acq Stopped)" {
            # "If we are waiting to stop, and the acquisition has already stopped, then the \"Logging Stopped\" message indicates that it is time to stop."
            n90 = call-poly "Enqueue Message.vi"("error in (no error)"=w302, "Message Data"="Ready..." ("Ready..."), "Message"="Update Status", "Message Queue"=w301) -> ("error out"=w300:errorcluster)  [unwired: 6 in, 1 out]
          }
        }
      }
      frame "Broadcast settings" {
        w313 = T33 {"Acq Settings"={"Instrument Specifications"=[], "Config Settings"={"Simulated Sensor Injection"=0.0, "Base Device Name"="", "Simulation Mode"=""}}, "Acquisition Context"={"Setpoint"=0.0, "Previous Setpoint"=0.0, "Transition Start Time"=0.0, "Transition Active?"=FALSE, "Acknowledgement Pending?"=FALSE}, "Stimulus Settings"={"Stimulus Outputs"=[]}}  # Acquisition Payload
        # "Broadcast settings - Send the 'Update Settings' message to the Acquisition message loop."
        n91 = Unbundle By Name(w307) -> ("Acq Settings"=w312:T12, "Test Sequence Settings.Test Sequence State.Current Target"=w311:dbl, "Test Sequence Settings.Test Sequence State.Previous Target"=w310:dbl, "Test Sequence Settings.Test Sequence State.Transition Active?"=w309:bool)
        n92 = Bundle By Name(cluster=w313, "Acq Settings"=w312, "Acquisition Context.Setpoint"=w311, "Acquisition Context.Previous Setpoint"=w310, "Acquisition Context.Transition Active?"=w309) -> (w308:T33)
        n93 = call-poly "Enqueue Message.vi"("error in (no error)"=w306, "Message Data"=w308, "Message"="Update Settings", "Message Queue"=w314) -> ("error out"=w316:errorcluster)  [unwired: 6 in, 1 out]
        n94 = Merge Errors(w316) -> (w320:errorcluster)
      }
      frame "Acquisition Settings Applied" {
        # "The Processing Loop resumes with waveforms running at the new setpoint, the updated \nTest Sequence Context (that is, direction and cycle number), and internal messages flushed from its queue."
        # "Acquisition Settings Applied - Send the 'Update Settings' message to the Processing message loop."
        n95 = call "Create Processing Payload.vi"("error in (no error)"=w330, "Settings in"=w329) -> ("error out"=w324:errorcluster, "Processing Settings"=w328:T16, "Settings out"=w327:T11)  [unwired: 7 in]
        n96 = Flush Queue(queue=w325, error in (no error)=w324) -> (error out=w323:errorcluster)  [unwired: 2 out]
        n97 = Flush Queue(queue=w321, error in (no error)=w323) -> (error out=w322:errorcluster)  [unwired: 2 out]
        n98 = call-poly "Enqueue Message.vi"("error in (no error)"=w322, "Message Data"=w328, "Message"="Update Settings", "Message Queue"=w321) -> ("error out"=w326:errorcluster)  [unwired: 6 in, 1 out]
        n99 = Merge Errors(w326) -> (w335:errorcluster)
      }
      frame "Launch Settings Dialog" {
        # "Launch Settings Dialog - Launch the Settings Dialog when the user clicks the 'Settings' button."
        n100 = call-by-ref "?"("Settings in"=w355, "Database in"=w356, "error in (no error)"=w358) -> ("Database out"=w337:refnum<queue>, "Settings out"=w352:T11, "UI Refresh Needed?"=w353:bool, "error out"=w339:errorcluster)  [unwired: 9 in, 4 out]
        n101 = Unbundle By Name(w352) -> ("Acq Settings.Instrument Specifications"=w340:T13)
        n102 = call "Remove Zeroes From Instrument Specs.vi"("error in (no error)"=w339, "Acq Settings.Instrument Specifications in"=w340) -> ("error out"=w338:errorcluster, "Acq Settings.Instrument Specifications out"=w336:T13)  [unwired: 8 in]
        n103 = case shown="True" w353 {
          tunnel: w338 -> [w360 w369]
          tunnel: [w360 w365] -> w346
          tunnel: w337 -> [_ w368]
          tunnel: [w359 w364] -> w349
          tunnel: w350 -> [_ w362]
          tunnel: w336 -> [_ w361]
          frame False {
            w359 = T1 []  # Sensor CoreData
          }
          frame True {
            n104 = for {
              tunnel: w368 -> [w375]
              tunnel: [w374] -> w367
              tunnel: [w371] -> w363 mode=indexing
              shift-right: [w373] -> w366
              shift-left: w369 -> [w376]
              tunnel: w361 -> [w370] mode=indexing
              n105 = Unbundle By Name(w370) -> ("Sensor ID *"=w372:i32)
              n106 = call "Fetch Sensor Data.vi"("error in (no error)"=w376, "SensorID"=w372, "Database"=w375) -> ("error out"=w373:errorcluster, "Data Valid?"=w374:bool, "Sensor CoreData Cluster"=w371:T2)  [unwired: 6 in]
            }
            n107 = case shown="True" w367 {
              tunnel: w366 -> [w378 w384]
              tunnel: [w378 w383] -> w365
              tunnel: [w377 w382] -> w364
              tunnel: w363 -> [_ w382]
              tunnel: w362 -> [_ w381]
              frame False {
                w377 = T1 []  # Sensor CoreData
                n108 = One Button Dialog(message="Error: The Database failed to return the\nSensor Profile. Please verify the Serial\nNumber or check the database connection.") -> ()  [unwired: 1 in, 1 out]
              }
              frame True {
                n109 = call-poly "Enqueue Message.vi"("error in (no error)"=w384, "Message"="Broadcast Settings", "Message Queue"=w381) -> ("error out"=w383:errorcluster)  [unwired: 7 in, 1 out]
              }
            }
          }
        }
        n110 = call "Remove Zeroes.vi"("error in (no error)"=w346, "Sensor Information in"=w349) -> ("error out"=w342:errorcluster, "Sensor Information out"=w348:T1)  [unwired: 8 in]
        "Sensor Information" <- w348
        n111 = Bundle By Name(cluster=w352, "Acq Settings.Instrument Specifications"=w336, "Processing Settings.Sensor CoreData"=w348) -> (w351:T11)
        n112 = Unbundle By Name(w345) -> ("Start Ref"=w344:refnum<vi>)
        n113 = Build Array(w344) -> (w343:refnum<vi>[])
        n114 = call "Set Enable State on Multiple Controls.vi"("Controls"=w343, "Disabled"=T32."Enabled", "error in (no error)"=w342) -> ("error out"=w341:errorcluster)  [unwired: 7 in]
      }
      frame "Launch Report Dialog" {
        # "Launch Settings Dialog - Launch the Settings Dialog when the user clicks the 'Settings' button."
        n115 = call-by-ref "?"("error in (no error)"=w391, "Database in"=w385) -> ("error IO"=w387:errorcluster)  [unwired: 10 in, 3 out]
      }
      frame "Manage Serial Numbers" {
        # "Manage Serial Numbers Dialog - Launch the Manage Serial Numbers Dialog when the user clicks the 'Manage Serial Numbers' button."
        n116 = call-by-ref "?"("Database"=w392, "error in (no error)"=w401, "System Config"=w395) -> ("error out"=w399:errorcluster)  [unwired: 9 in, 3 out]
        n117 = call-poly "Enqueue Message.vi"("error in (no error)"=w399, "Message"="Broadcast Settings", "Message Queue"=w400) -> ("error out"=w396:errorcluster)  [unwired: 7 in, 1 out]
      }
      frame "Error" {
        # "Error - Display an error dialog. This message is sent by the \"Error Handler\" VIs at the end of other loops in this application."
        n118 = Variant To Data(error in=w403, type=errorcluster {"status"=FALSE, "code"=0, "source"=""} ("error constant"), Variant=w407) -> (data=w404:errorcluster, error out=w408:errorcluster)
        n119 = call <vilib>:"Simple Error Handler.vi"("error in (no error)"=w404) -> ()  [unwired: 4 in, 5 out]
        n120 = Merge Errors(w408) -> (w406:errorcluster)
      }
      frame "Confirm Quit" {
        # "Confirm Quit - Message that can confirm whether or not the user wants to exit the application."
        n121 = case shown="\"Acquiring and Logging\"" w417 {
          tunnel: w416 -> [w425 w429]
          tunnel: w415 -> [w424 w428]
          tunnel: [w423 w427] -> w414
          tunnel: [UI_State."Idle" ("UI State") w426] -> w413
          frame Default {
            # "If 'Confirm Quit' comes in while the system is idle, there is no need for a confirmation message."
            n122 = call-poly "Enqueue Message.vi"("Priority Message? (F)"=TRUE, "error in (no error)"=w424, "Message"="Exit", "Message Queue"=w425) -> ("error out"=w423:errorcluster)  [unwired: 6 in, 1 out]
          }
          frame "Acquiring and Logging" {
            n123 = Two Button Dialog(message="Are you sure you want to quit while the acquisition is running?" ("Confirm Quit Message"), 1:"No" ("No"), 2:"Yes" ("Yes")) -> (T button?=w430:bool)
            n124 = case shown="True" w430 {
              tunnel: w429 -> [_ w439]
              tunnel: w428 -> [w435 w440]
              tunnel: [w435 w438] -> w427
              tunnel: [UI_State."Acquiring and Logging" ("UI State") UI_State."Waiting for Exit" ("UI State")] -> w426
              frame False {
                # "User did not want to quit."
              }
              frame True {
                n125 = call-poly "Enqueue Message.vi"("error in (no error)"=w440, "Message"="Stop", "Message Queue"=w439) -> ("error out"=w438:errorcluster)  [unwired: 7 in, 1 out]
              }
            }
          }
        }
      }
      frame "Exit" {
        w443 = TRUE ("Priority Message? (F)")
        w442 = "Exit" ("Message")
        # "Popup an error dialog if 'Exit' was called as a result of an error."
        # "Stop the VI"
        # "Exit - Send Exit messages to the Acquisition and Logging loops, and fire the user event to stop the Event Handling Loop."
        n126 = call-poly "Enqueue Message.vi"("Priority Message? (F)"=w443, "error in (no error)"=w447, "Message"=w442, "Message Queue"=w450) -> ("error out"=w448:errorcluster)  [unwired: 6 in, 1 out]
        n127 = Variant To Data(type=errorcluster {"status"=FALSE, "code"=0, "source"=""} ("error constant"), Variant=w452) -> (data=w451:errorcluster)  [unwired: 1 in, 1 out]
        n128 = call <vilib>:"Simple Error Handler.vi"("error in (no error)"=w451) -> ()  [unwired: 4 in, 5 out]
        n129 = call-poly "Enqueue Message.vi"("Priority Message? (F)"=w443, "error in (no error)"=w448, "Message"=w442, "Message Queue"=w449) -> ("error out"=w454:errorcluster)  [unwired: 6 in, 1 out]
        n130 = call-poly "Enqueue Message.vi"("Priority Message? (F)"=w443, "error in (no error)"=w454, "Message"=w442, "Message Queue"=w456) -> ("error out"=w445:errorcluster)  [unwired: 6 in, 1 out]
        n131 = call-poly "Enqueue Message.vi"("Priority Message? (F)"=w443, "error in (no error)"=w445, "Message"=w442, "Message Queue"=w441) -> ("error out"=w444:errorcluster)  [unwired: 6 in, 1 out]
        n132 = call "Fire User Event - Stop.vi"("error in (no error)"=w444, "User Event - Stop"=w460) -> ("error out"=w459:errorcluster)  [unwired: 9 in]
      }
      frame "---Copy This Frame---" {
        # "Duplicate this frame when creating new messages.  Change this comment in the duplicated frame to describe this message."
        n133 = Merge Errors(w467) -> (w466:errorcluster)
      }
      frame Default {
        # "'Default' case only runs if there is a message that isn't defined in any of the other cases.  Output a programming error."
        n134 = xnode "Error Ring"("parameter 0"=w470) -> ("error out"=w469:errorcluster)
      }
    }
    n135 = call "Error Handler - Message Handling Loop.vi"("error in (no error)"=w94, "Message Queue"=w93) -> ("dup error in"=w95:errorcluster)  [unwired: 8 in, 1 out]
  }
  n136 = call "Processing Message Loop.vi"("error in (no error)"=w2, "Queue A - Processing"=w10, "Message Queues"=w6) -> ("error out"=w18:errorcluster)  [unwired: 8 in]
  n137 = call "Logging Message Loop.vi"("error in (no error)"=w2, "Queue B -TDMS Raw"=w11, "Message Queues"=w6) -> ("error out"=w39:errorcluster)  [unwired: 8 in]
  n138 = Wait on Notification(notifier=w4, error in (no error)=w2) -> (notification=w8:T5, error out=w1:errorcluster)  [unwired: 2 in, 2 out]
  n139 = Unbundle By Name(w8) -> ("SensorIDs"=w5:i32[])
  n140 = for {
    tunnel: w5 -> [w489] mode=indexing
    tunnel: w7 -> [w488]
    shift-right: [w484] -> w3
    shift-left: w1 -> [w485]
    i -> [w492]
    n141 = call "Fetch Sensor Data.vi"("error in (no error)"=w485, "SensorID"=w489, "Database"=w488) -> ("error out"=w486:errorcluster, "Sensor CoreData Cluster"=w487:T2)  [unwired: 6 in, 1 out]
    n142 = control-ref of="Data"() -> (w483:refnum<vi>)
    n143 = property class="WFChart (strict)"(reference=w483, error in=w486, "Active Plot"=w492) -> (reference out=w491:refnum<vi>, error out=w490:errorcluster)
    n144 = Unbundle By Name(w487) -> ("SerialNumber"=w482:string)
    n145 = Concatenate Strings("SN: " ("string"), w482) -> ()  [unwired: 1 out]
    n146 = property class="WFChart (strict)"(reference=w491, error in=w490, "Plot.Plot Name"=w482) -> (error out=w484:errorcluster)  [unwired: 1 out]
  }
  n147 = while "Data Display Loop" {
    tunnel: w4 -> [w497]
    tunnel: w6 -> [_]
    tunnel: w3 -> [w493]
    stop <- w494 stop-if-true
    # "Data Display Loop"
    n148 = Wait on Notification(notifier=w497, error in (no error)=w493) -> (notification=w496:T5, error out=w494:errorcluster)  [unwired: 2 in, 2 out]
    n149 = call "Convert Signal to Engineering Units.vi"() -> ()  [unwired: 10 in, 2 out]
    n150 = Unbundle By Name(w496) -> ("Waveforms"=→"Data":waveform(dbl)[])
  }
  n151 = Unregister For Events(event registration refnum=w36, error in=w42) -> (error out=w37:errorcluster)
  n152 = Release Queue(queue=w30, error in (no error)=w43) -> (error out=w28:errorcluster)  [unwired: 1 in, 2 out]
  n153 = Release Queue(queue=w10, error in (no error)=w28) -> (error out=w13:errorcluster)  [unwired: 1 in, 2 out]
  n154 = Release Queue(queue=w11, error in (no error)=w13) -> (error out=w12:errorcluster)  [unwired: 1 in, 2 out]
  n155 = Release Notifier(notifier=w4, error in (no error)=w12) -> (error out=w27:errorcluster)  [unwired: 1 in, 2 out]
  n156 = Merge Errors(w37, w27, w41, w39, w22, w18) -> (w31:errorcluster)
  n157 = call "Destroy User Event - Stop.vi"("error in (no error)"=w31, "User Event - Stop"=w25) -> ("error out"=w29:errorcluster)  [unwired: 9 in]
  n158 = disable-structure shown="RUN_TIME_ENGINE==True" {
    disable-tunnel: w29 -> [_ _]
    frame condition #0 (active) {
    }
    frame condition #1 {
      # "Call Quit LabVIEW if running as a built application."
      n159 = Quit LabVIEW() -> ()  [unwired: 1 in]
    }
  }
